vi "NI VeriStand - Close Stimulus Profile Manager Reference.vi"(8 "error in (no error)":errorcluster, 11 "StimulusProfileManager":T1) -> (0 "error out":errorcluster)   [LabVIEW 2020, in "NI_VS Stimulus ExecutionAPI.lvlib"]
doc: "This VI interfaces with the legacy Stimulus Profile Editor workspace tool in NI VeriStand, and is included for compatibility only. National Instruments recommends you use the current Stimulus Profile VIs to create, observe, and control NI VeriStand stimulus profiles and real-time sequences.\n\nCloses an open reference to the stimulus profile manager on the VeriStand Gateway. Use this VI to close each stimulus profile manager reference that you open with the Open Stimulus Profile Manager VI."
uses:
  <vilib>/NI VeriStand/Execution/Stimulus/NI_VS Stimulus ExecutionAPI.lvlib
  <vilib>/NI VeriStand/Execution/Stimulus/StimulusAPI.ctl
  NationalInstruments.VeriStand.ClientAPI
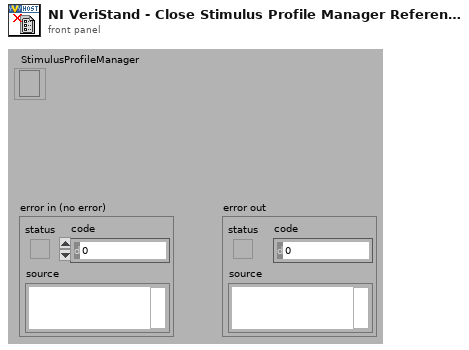
[diagram p1: front panel]
types:
  T1 = typedef "NI_VS Stimulus ExecutionAPI.lvlib/StimulusAPI.ctl" = refnum<k24>
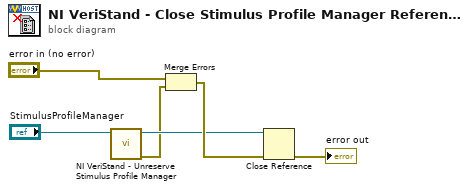
[diagram p0: block diagram]
diagram:
  n1 = call <vilib>:"NI VeriStand - Unreserve Stimulus Profile Manager.vi"("StimulusProfileManager in"="StimulusProfileManager") -> ("error out"=w1:errorcluster, "StimulusProfileManager out"=w3:T1)  [unwired: 1 in, 8 out]
  n2 = Merge Errors("error in (no error)", w1) -> (w5:errorcluster)
  n3 = Close Reference(reference=w3, error in (no error)=w5) -> (error out=→"error out":errorcluster)
